vi "NavXGyroCalc.vi"(11 "Button Input":bool) -> (3 "Yaw":dbl)   [LabVIEW 2018]
uses:
  <vilib>/Rock Robotics/Network Tables/NT Write Boolean.vi
  <vilib>/Rock Robotics/Network Tables/NT Write Number.vi
panel:
  out "YRPHfH":T1
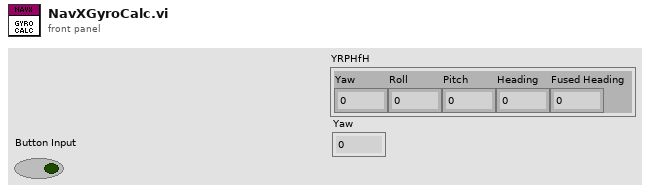
[diagram p1: front panel]
types:
  T1 = cluster{"Yaw":dbl, "Roll":dbl, "Pitch":dbl, "Heading":dbl, "Fused Heading":dbl}
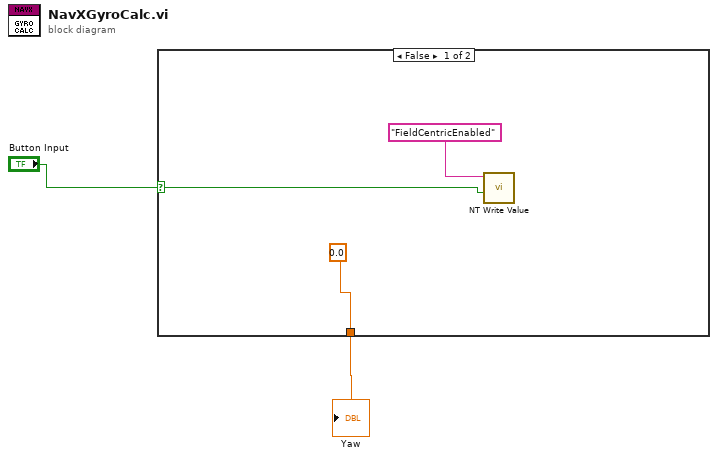
[diagram p0: block diagram]
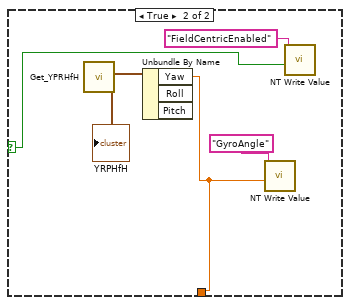
[diagram p2: hidden frame]
diagram:
  n1 = case shown="False" "Button Input" {
    selector: "Button Input" -> [w4 w8]
    tunnel: [0.0 ("Yaw") w6] -> w1
    frame False {
      n2 = call-poly <vilib>:"NT Write Value.vi"("Boolean"=w4, "Name"="FieldCentricEnabled") -> ()  [unwired: 9 in, 1 out]
    }
    frame True {
      n3 = call <vilib>:"Get_YPRHfH.vi"() -> ("YRPHfH"=w10:T1)  [unwired: 11 in]
      "YRPHfH" <- w10
      n4 = Unbundle By Name(w10) -> ("Yaw"=w6:dbl)  [unwired: 2 out]
      n5 = call-poly <vilib>:"NT Write Value.vi"("Numeric"=w6, "Name"="GyroAngle") -> ()  [unwired: 9 in, 1 out]
      n6 = call-poly <vilib>:"NT Write Value.vi"("Boolean"=w8, "Name"="FieldCentricEnabled") -> ()  [unwired: 9 in, 1 out]
    }
  }
  "Yaw" <- w1
